vi "Dashboard Main.vi"() -> ()   [LabVIEW 2013]
uses:
  <vilib>/event_ctls.llb/eventvkey.ctl
  <vilib>/Rock Robotics/WPI/Dashboard/WPI_DashboardLogging Global.vi
  <vilib>/Utility/config.llb/Write Key (String).vi
  <vilib>/Utility/config.llb/Write Key (I32).vi
  <vilib>/Utility/config.llb/NI_LVConfig.lvlib
panel:
  out "Image Message":string="Timeout in Camera Communications"
  in  "Rec Mode":enum32{"Stop", "Record", "Playback"}(radio)
  in  "Dashboard Tab":T1(tab)
  in  "Camera Settings":T2={"Frame Rate"=30, "Compression"=30, "Size"=1} {"Frame Rate" scale=1.0..30.0; "Size" items=["640x480", "320x240", "160x120"]}
  out "MotorSliders R":cluster{"MotorSlide1":dbl, "MotorSlide2":dbl} {"MotorSlide2" scale=-1.0..1.0 scale format="%#_2e"; "MotorSlide1" scale=-1.0..1.0 scale format="%#_2e"}
  out "MotorChart R":cluster{"Numeric":dbl, "Numeric":dbl}(graph)
  out "MotorSliders L":T3 {"MotorSlide4 2" scale=0.0..14.0 scale format="%#_2e"; "MotorSlide2" scale=-1.0..1.0 scale format="%#_2e"; "MotorSlide1" scale=-1.0..1.0 scale format="%#_2e"}
  out "MotorChart L":T4(graph)
  out "JS1 Z":dbl(slide) scale=-1.0..1.0 scale format="%#_2e"
  out "Joystick 1":cluster{"X":dbl, "Y":dbl}[](graph)
  out "JS Buttons 1":T5
  out "JS2 Z":dbl(slide) scale=-1.0..1.0 scale format="%#_2e"
  out "Joystick 2":cluster{"X":dbl, "Y":dbl}[](graph)
  out "JS Buttons 2":T5
  out "Mode":T6(ring)=enum."Auto Disabled"
  out "Camera IP":string
  in  "DB Camera Config":bool
  out "fps":dbl format="%#.1g"
  out "Mbps":dbl format="%#.1g"
  out "Mbps 2":bool
  out "LED 1":bool
  out "Tanks Full":bool
  in  "Compressor On":bool
  out "Compression Pressure":dbl(slide) scale=0.0..10.0
  in  "Slider 1":dbl(slide) scale=0.0..100.0
  in  "Checkbox 2":bool
  in  "Checkbox 1":bool
  in  "Test Slider":dbl(slide) scale=0.0..100.0 scale format="%#_3g"
  in  "On/Off":bool caption="Solenoid"
  in  "Test Name":u16(ring) items=["Select the test to run...", "Example Test", "-------------------------------", "List of tests is built in robot code.", "Replace with your own automated tests."]
  in  "Test Tree":string(tree)
  in  "Motor":cluster{"Value":dbl, "Enable":bool} {"Value" scale=-1.0..1.0 scale format="%#_3g"}
  out "Progress":T7 {"Test Progress" scale=0.0..100.0}
  in  "Rev/Fwd":cluster{"Forward":bool, "Reverse":bool}
  in  "Test Ring":u16(ring) items=["Auto", "Fixed indoor", "Fixed outdoor 1", "Fixed outdoor 2", "Fixed fluorescent 1", "Fixed fluorescent 2", "Hold current"]
  in  "Listbox":i32(listbox)
  out "Tree":string(tree)
  out "Camera Image":T8(plugin-control)
  in  "Enable":bool
  # "Left"
  # "Front"
  # "Right"
  # "Battery"
  # "Customize by placing controls and indicators here and name to\nmatch Dashboard Variables on robot."
  # "This tab is a great place for autonomous settings and validation.\nCustomize by placing controls and indicators here and name to\nmatch Dashboard Variables on robot."
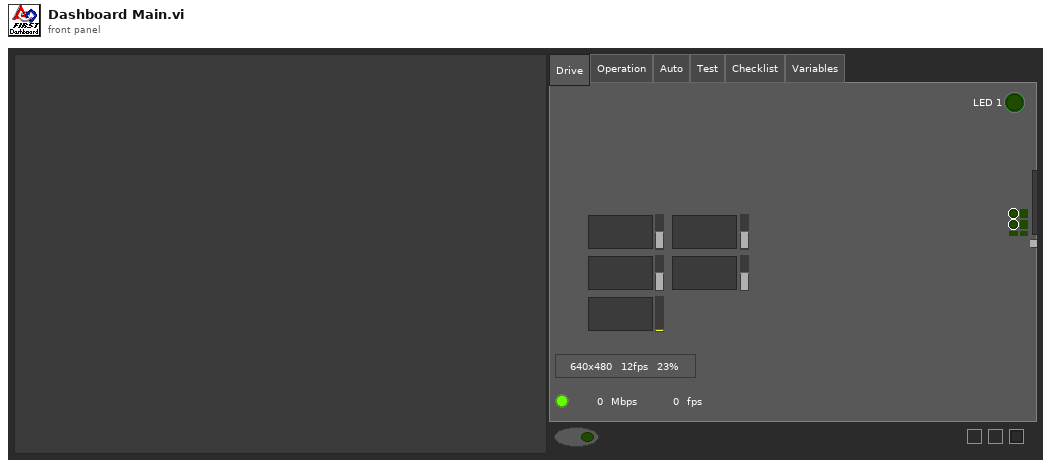
[diagram p1: front panel]
types:
  T1 = enum32{"Drive", "Operation", "Auto", "Test", "Checklist", "Variables"}
  T2 = cluster{"Frame Rate":i32, "Compression":i32, "Size":u16}
  T3 = cluster{"MotorSlide1":dbl, "MotorSlide2":dbl, "MotorSlide4 2":dbl}
  T4 = cluster{"Numeric":dbl, "Numeric":dbl, "Battery":sgl}
  T5 = cluster{bool, bool, bool, bool, bool, bool, bool, bool, bool, bool, bool, bool}
  T6 = enum8{"Tele-Op Disabled", "Tele-Op Enabled", "Auto Disabled", "Auto Enabled", "Test Disabled", "Test Enabled", ""}
  T7 = cluster{"Test Progress":u8, "Test Progress Text":string}
  T8 = typedef "IMAQ Image.ctl" = refnum<image>
  T9 = typedef "Image Type" = u32
  T10 = cluster{"Digital Inputs":bool[], "Digital Outputs":bool[]}
  T11 = cluster{"Competition mode":bool, "Robot Link":bool, "Autonomous":bool, "Enabled":bool, "E-Stop":bool, "Simulated":bool, "TestMode":bool, "Docked Window":bool}
  T12 = cluster{"Boolean Array[0]":bool, "Boolean Array[1]":bool, "Boolean Array[2]":bool, "Boolean Array[3]":bool, "Boolean Array[4]":bool, "Boolean Array[5]":bool, "Boolean Array[6]":bool, "Boolean Array[7]":bool, "Boolean Array[8]":bool, "Boolean Array[9]":bool, "Boolean Array[10]":bool, "Boolean Array[11]":bool}
  T13 = typedef "NI_LVConfig.lvlib/Config Data RefNum.ctl" = refnum<k1>
  T14 = typedef "eventvkey.ctl" = enum16{"ASCII", "Enter", "Return", "Shift", "Ctrl", "Alt", "Cmd", "Opt", "Caps", "NumLock", "Clear", "Break", "Up", "Down", "Left", "Right", "Insert", "Delete", "Home", "End", "PageUp", "PageDown", "Escape", "Help", "Pause", "ScrollLock", "F1", "F2", "F3", "F4", "F5", "F6", "F7", "F8", "F9", "F10", "F11", "F12", "F13", "F14", "F15", "F16", "F17", "F18", "F19", "F20", "F21", "F22", "F23", "F24", "Play", "VolumeUp", "VolumeDown", "Mute", "Two Byte Char"}
  T15 = cluster{"Image Size":bool, "Image Type":bool, "Pixel Value":bool, "ROI Information":bool, "Zoom Factor":bool}
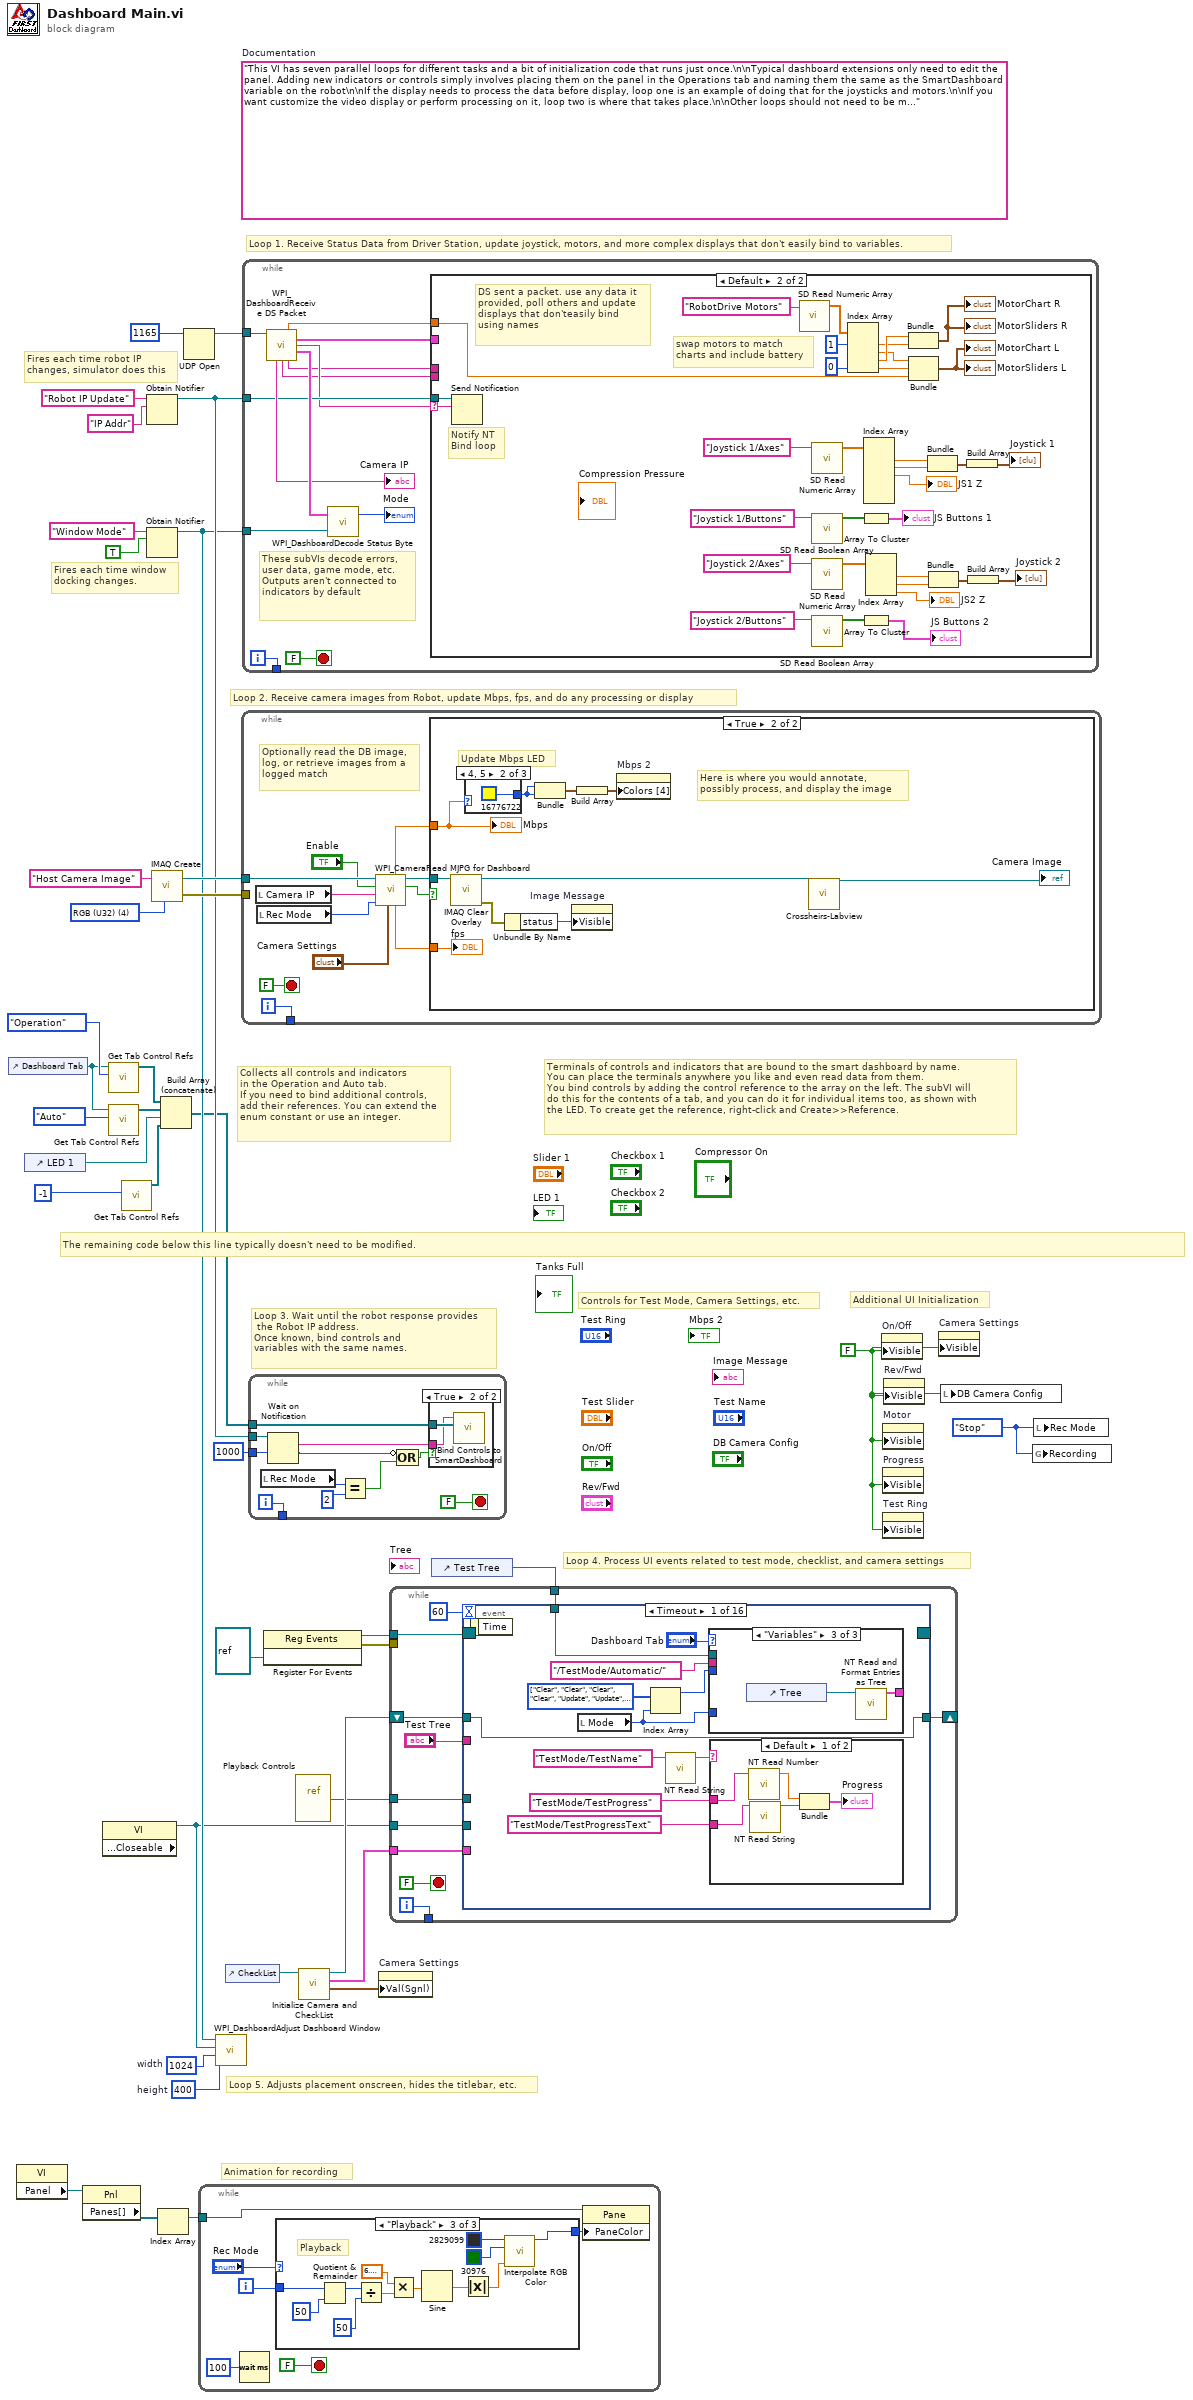
[diagram p0: block diagram]
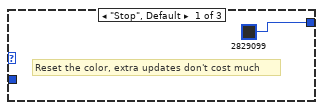
[diagram p2: hidden frame]
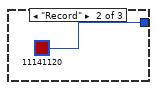
[diagram p3: hidden frame]
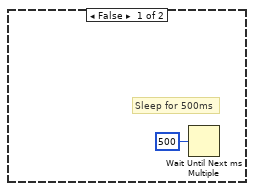
[diagram p5: hidden frame]
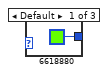
[diagram p6: hidden frame]
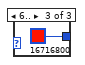
[diagram p7: hidden frame]
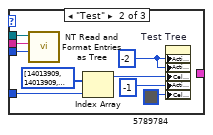
[diagram p9: hidden frame]
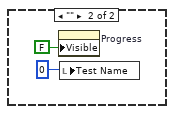
[diagram p10: hidden frame]
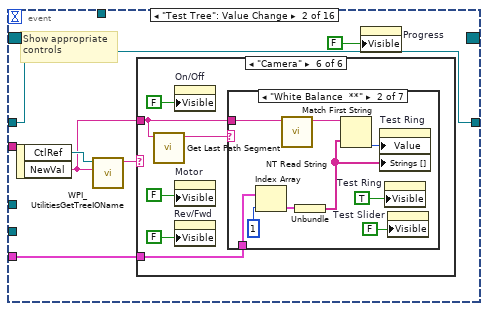
[diagram p11: hidden frame]
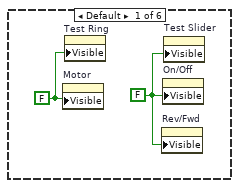
[diagram p12: hidden frame]
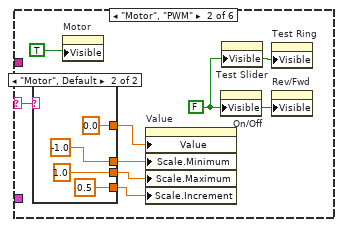
[diagram p13: hidden frame]
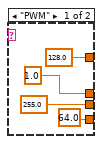
[diagram p14: hidden frame]
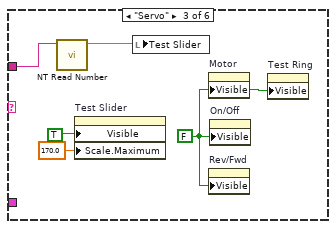
[diagram p15: hidden frame]
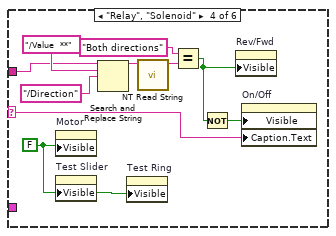
[diagram p16: hidden frame]
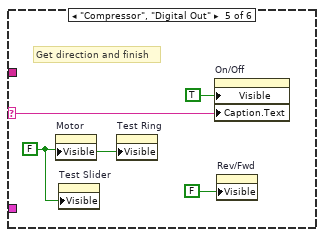
[diagram p17: hidden frame]
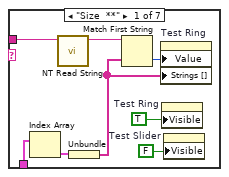
[diagram p18: hidden frame]
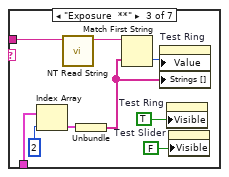
[diagram p19: hidden frame]
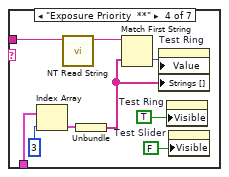
[diagram p20: hidden frame]
diagram:
  w10 = enum32{"Stop", "Record", "Playback"}."Stop" ("Rec Mode")
  w13 = 400  # height
  w14 = 1024  # width
  w27 = FALSE ("Visible")
  (unwired) "This VI has seven parallel loops for different tasks and a bit of initialization code that runs just once.\n\nTypical dashboard extensions only need to edit the panel. Adding new indicators or controls simply involves placing them on the panel in the Operations tab and naming them the same as the SmartDashboard variable on the robot\n\nIf the display needs to process the data before display, loop one is an example of doing that for the joysticks and motors.\n\nIf you want customize the video display or perform processing on it, loop two is where that takes place.\n\nOther loops should not need to be modified. They are pretty standard, and document the task they perform."  # Documentation
  w37 = T9 4 items=["Grayscale (U8)", "Grayscale (I16)", "Grayscale (SGL)", "Complex (CSG)", "RGB (U32)", "HSL (U32)", "RGB (U64)"] ("Image Type")
  # "Controls for Test Mode, Camera Settings, etc."
  # "Additional UI Initialization"
  # "Animation for recording"
  # "Fires each time robot IP\nchanges, simulator does this"
  # "Fires each time window\ndocking changes."
  # "Collects all controls and indicators\nin the Operation and Auto tab.\nIf you need to bind additional controls,\nadd their references. You can extend the\nenum constant or use an integer."
  # "The remaining code below this line typically doesn't need to be modified."
  # "Loop 4. Process UI events related to test mode, checklist, and camera settings"
  # "Terminals of controls and indicators that are bound to the smart dashboard by name.\nYou can place the terminals anywhere you like and even read data from them.\nYou bind controls by adding the control reference to the array on the left. The subVI will\ndo this for the contents of a tab, and you can do it for individual items too, as shown with\nthe LED. To create get the reference, right-click and Create>>Reference."
  # "Loop 3. Wait until the robot response provides\n the Robot IP address.\nOnce known, bind controls and\nvariables with the same names."
  # "Loop 5. Adjusts placement onscreen, hides the titlebar, etc."
  # "Loop 1. Receive Status Data from Driver Station, update joystick, motors, and more complex displays that don't easily bind to variables."
  # "Loop 2. Receive camera images from Robot, update Mbps, fps, and do any processing or display"
  n1 = control-ref of="Dashboard Tab"() -> (w8:refnum<vi>)
  n2 = property class="VI"() -> ("Panel"=w21:refnum<vi>)  [unwired: 2 in, 2 out]
  n3 = control-ref of="LED 1"() -> (w3:refnum<vi>)
  n4 = property class="Pnl"(reference=w21) -> ("Panes[]"=w22:refnum<vi>[])  [unwired: 1 in, 2 out]
  n5 = property class="VI" props=["Front Panel.Closeable"]() -> (reference out=w9:refnum<vi>)  [unwired: 2 in, 2 out]
  n6 = call <vilib>:"Get Tab Control Refs.vi"("Page Index"=T1."Operation" ("Dashboard Tab"), "TabControl in"=w8) -> ("ControlsOnPage"=w6:refnum<vi>[])  [unwired: 9 in]
  n7 = call <vilib>:"Get Tab Control Refs.vi"("Page Index"=T1."Auto" ("Dashboard Tab"), "TabControl in"=w8) -> ("ControlsOnPage"=w7:refnum<vi>[])  [unwired: 9 in]
  n8 = call <vilib>:"Get Tab Control Refs.vi"("Page Index"=-1) -> ("ControlsOnPage"=w2:refnum<vi>[])  [unwired: 10 in]
  n9 = Obtain Notifier(name (unnamed)="Robot IP Update", notification data type="IP Addr" ("name (unnamed)")) -> (notifier out=w31:refnum<notifier>)  [unwired: 2 in, 2 out]
  n10 = Obtain Notifier(name (unnamed)="Window Mode", notification data type=TRUE) -> (notifier out=w12:refnum<notifier>)  [unwired: 2 in, 2 out]
  n11 = call "IMAQ Create"("Image Name"="Host Camera Image", "Image Type"=w37) -> ("New Image"=w35:T8, "error out"=w34:errorcluster)  [unwired: 2 in, 1 out]
  n12 = Index Array(array=w22) -> (element=w20:refnum<vi>)  [unwired: 1 in]
  n13 = Build Array (concatenate)(w6, w7, w3, w2) -> (w5:refnum<vi>[])
  n14 = UDP Open(11:u16 1165 ("port")) -> (port=w38:refnum<k16>)  [unwired: 2 in, 4 out]
  n15 = while {
    tunnel: w20 -> [w41]
    i -> [w44]
    stop <- FALSE stop-if-true
    n16 = Wait (ms)(milliseconds to wait=u32 100) -> ()  [unwired: 1 out]
    n17 = case shown="\"Playback\"" "Rec Mode" {
      tunnel: w44 -> [_ _ w59]
      tunnel: [u32 2829099 ("Base Color") u32 11141120 ("Target Color") w48] -> w40
      frame "Stop", Default {
        # "Reset the color, extra updates don't cost much"
      }
      frame "Record" {
      }
      frame "Playback" {
        # "Playback"
        n18 = Quotient & Remainder(x=w59, y=u32 50 ("milliseconds to wait")) -> (x-y*floor(x/y)=w55:u32)  [unwired: 1 out]
        n19 = Divide(x=w55, y=u32 50 ("milliseconds to wait")) -> (x/y=w52:dbl)
        n20 = Multiply(x=6.283185307179586, y=w52) -> (x*y=w57:dbl)
        n21 = Sine(x=w57) -> (sin(x)=w56:dbl)
        n22 = Absolute Value(x=w56) -> (abs(x)=w49:dbl)
        n23 = call "Interpolate RGB Color.vi"("Proportion"=w49, "Target Color"=u32 30976, "Base Color"=u32 2829099) -> ("Result Color"=w48:u32)  [unwired: 8 in]
      }
    }
    n24 = property class="Pane"(reference=w41, "PaneColor"=w40) -> ()  [unwired: 1 in, 2 out]
  }
  n25 = call <vilib>:"WPI_DashboardAdjust Dashboard Window.vi"("height"=w13, "width"=w14, "reference in"=w9, "Notifier in"=w12) -> ()  [unwired: 8 in]
  n26 = control-ref of="CheckList"() -> (w11:refnum<vi>)
  n27 = while {
    tunnel: w35 -> [w68]
    tunnel: w34 -> [_]
    tunnel: [w69] -> _
    i -> [w69]
    stop <- FALSE stop-if-true
    # "Optionally read the DB image,\nlog, or retrieve images from a\nlogged match"
    n28 = local read "Camera IP"() -> (w61:string)
    n29 = local read "Rec Mode"() -> (w60:enum32{"Stop", "Record", "Playback"})
    n30 = call <vilib>:"WPI_CameraRead MJPG for Dashboard.vi"("Camera Settings"="Camera Settings", "Rec Mode"=w60, "Camera IP"=w61, "Enable"="Enable", "Refnum in"=w68) -> ("Active"=w65:bool, "Refnum out"=w67:T8, "FPS"=w64:dbl, "Bandwidth (Mbps)"=w63:dbl)  [unwired: 3 in]
    n31 = case shown="True" w65 {
      tunnel: w67 -> [_ w76]
      tunnel: w63 -> [_ w75]
      tunnel: w64 -> [_ w74]
      frame False {
        # "Sleep for 500ms"
        n32 = Wait Until Next ms Multiple(millisecond multiple=u32 500) -> ()  [unwired: 1 out]
      }
      frame True {
        # "Here is where you would annotate,\npossibly process, and display the image"
        # "Update Mbps LED"
        n33 = call "IMAQ Clear Overlay"("Image"=w76) -> ("error out"=w80:errorcluster, "Image Out"=w73:T8)  [unwired: 2 in, 7 out]
        n34 = case shown="4, 5" w75 {
          tunnel: [u32 6618880 ("Color Box") u32 16776722 ("Color Box") u32 16716800 ("Color Box")] -> w77
          frame Default {
          }
          frame 4, 5 {
          }
          frame 6.. {
          }
        }
        n35 = Unbundle By Name(w80) -> ("status"=w81:bool)
        n36 = Bundle("Color Box"=w77, "Color Box"=w77) -> (w79:cluster{"Color Box":u32, "Color Box":u32})  [unwired: 1 out]
        n37 = property on="Image Message" class="Str"("Visible"=w81) -> ()  [unwired: 2 in, 2 out]
        n38 = Build Array(w79) -> (w78:cluster{"Color Box":u32, "Color Box":u32}[])
        n39 = property on="Mbps 2" class="Bool (strict)"("Colors [4]"=w78) -> ()  [unwired: 2 in, 2 out]
        n40 = call "Crossheirs-Labview.vi"("Image In"=w73) -> ("Image Out"=→"Camera Image":T8)  [unwired: 25 in, 1 out]
        "Mbps" <- w75
        "fps" <- w74
      }
    }
  }
  n41 = while {
    tunnel: w38 -> [w95]
    tunnel: w31 -> [w90]
    tunnel: w12 -> [w94]
    tunnel: [w91] -> _
    i -> [w91]
    stop <- FALSE stop-if-true
    # "These subVIs decode errors, user data, game mode, etc.\nOutputs aren't connected to indicators by default"
    n42 = call <vilib>:"WPI_DashboardReceive DS Packet.vi"("Recv Socket"=w95) -> ("Battery"=w85:sgl, "Driver Station"=w86:T10, "Robot IP Address"=w89:string, "Status"=w96:T11, "Camera IP Address"=→"Camera IP":string, "Low Priority User Data"=w88:string, "High Priority User Data"=w87:string)  [unwired: 1 in, 7 out]
    n43 = call <vilib>:"WPI_DashboardDecode Status Byte.vi"("Window Mode Notifier"=w94, "Status"=w96) -> ("Mode"=→"Mode":T6)  [unwired: 1 out]
    n44 = case shown="Default" w89 {
      selector: w89 -> [_ w108]
      tunnel: w90 -> [_ w109]
      tunnel: w88 -> [_ _]
      tunnel: w87 -> [_ _]
      tunnel: w86 -> [_ _]
      tunnel: w85 -> [_ w107]
      frame "0.0.0.0" {
        # "DS not sending packets, or no robot exists yet.\nDon't poll the variables"
      }
      frame Default {
        # "Notify NT\nBind loop"
        # "DS sent a packet. use any data it\nprovided, poll others and update\ndisplays that don'teasily bind\nusing names"
        # "swap motors to match\ncharts and include battery"
        n45 = Send Notification(notification=w108, notifier=w109) -> ()  [unwired: 1 in, 2 out]
        n46 = call <vilib>:"SD Read Numeric Array.vi"("Name"="RobotDrive Motors") -> ("Numeric Array"=w106:dbl[])  [unwired: 8 in, 2 out]
        n47 = call <vilib>:"SD Read Numeric Array.vi"("Name"="Joystick 1/Axes") -> ("Numeric Array"=w125:dbl[])  [unwired: 8 in, 2 out]
        n48 = call <vilib>:"SD Read Boolean Array.vi"("Name"="Joystick 1/Buttons") -> ("Boolean Array"=w127:bool[])  [unwired: 8 in, 2 out]
        n49 = call <vilib>:"SD Read Numeric Array.vi"("Name"="Joystick 2/Axes") -> ("Numeric Array"=w119:dbl[])  [unwired: 8 in, 2 out]
        n50 = call <vilib>:"SD Read Boolean Array.vi"("Name"="Joystick 2/Buttons") -> ("Boolean Array"=w118:bool[])  [unwired: 8 in, 2 out]
        n51 = Index Array(array=w106, index #1=1, index #4=0) -> (element #1=w102:dbl, element #2=w101:dbl, element #3=w103:dbl, element #4=w98:dbl)  [unwired: 2 in]
        n52 = Array To Cluster(array=w127) -> (cluster=→"JS Buttons 1":T12)
        n53 = Array To Cluster(array=w118) -> (cluster=→"JS Buttons 2":T12)
        n54 = Index Array(array=w125) -> (element #1=w122:dbl, element #2=w123:dbl, element #3=→"JS1 Z":dbl)  [unwired: 6 in, 3 out]
        n55 = Index Array(array=w119) -> (element #1=w114:dbl, element #2=w113:dbl, element #3=→"JS2 Z":dbl)  [unwired: 3 in]
        n56 = Bundle("Numeric"=w103, "Numeric"=w102) -> (→"MotorChart R" →"MotorSliders R":cluster{"Numeric":dbl, "Numeric":dbl})  [unwired: 1 in]
        n57 = Bundle("Numeric"=w101, "Numeric"=w98, "Battery"=w107) -> (→"MotorChart L" →"MotorSliders L":T4)  [unwired: 1 in]
        n58 = Bundle("Numeric"=w122, "Numeric"=w123) -> (w121:cluster{"Numeric":dbl, "Numeric":dbl})  [unwired: 1 in]
        n59 = Bundle("Numeric"=w114, "Numeric"=w113) -> (w115:cluster{"Numeric":dbl, "Numeric":dbl})  [unwired: 1 in]
        n60 = Build Array(w121) -> (→"Joystick 1":cluster{"Numeric":dbl, "Numeric":dbl}[])
        n61 = Build Array(w115) -> (→"Joystick 2":cluster{"Numeric":dbl, "Numeric":dbl}[])
      }
    }
  }
  n62 = while {
    tunnel: w5 -> [w141]
    tunnel: w31 -> [w139]
    tunnel: [w137] -> _
    tunnel: u32 1000 ("milliseconds to wait") -> [w136]
    i -> [w137]
    stop <- FALSE stop-if-true
    n63 = local read "Rec Mode"() -> (w132:enum32{"Stop", "Record", "Playback"})
    n64 = Wait on Notification(notifier=w139, timeout in ms (-1)=w136) -> (notification=w138:string, timed out?=w134:bool)  [unwired: 2 in, 2 out]
    n65 = Equal?(x=w132, y=u16 2 ("Rec Mode")) -> (x = y?=w133:bool)
    n66 = Compound Arithmetic op=OR(invert w134, w133) -> (w135:bool)
    n67 = case shown="True" w135 {
      tunnel: w141 -> [_ w143]
      tunnel: w138 -> [_ w142]
      frame False {
      }
      frame True {
        n68 = call <vilib>:"Bind Controls to SmartDashboard.vi"("Bound Control Refs"=w143, "Server IP Address"=w142) -> ()  [unwired: 10 in]
      }
    }
  }
  n69 = register-events(refnum<vi> refnum) -> (reference out=w18:refnum<event-registration>, error out=w17:errorcluster)  [unwired: 2 in]
  n70 = vi-ref "Playback Controls.vi"() -> (w19:refnum<vi>)
  n71 = call "Initialize Camera and CheckList.vi"("ListBox in"=w11) -> ("Cluster"=w25:cluster{"value":i32, "value":i32, "index":i32}, "Array"=w26:cluster{string[]}[], "File Refnum"=w24:T13)  [unwired: 8 in]
  n72 = property on="Camera Settings" class="Clust (strict)"("Val(Sgnl)"=w25) -> ()  [unwired: 2 in, 2 out]
  n73 = control-ref of="Test Tree"() -> (w23:refnum<vi>)
  n74 = while {
    tunnel: w26 -> [w151]
    shift-right: [w150] -> _
    shift-left: w24 -> [w149]
    tunnel: [w148] -> _
    tunnel: w23 -> [w147]
    tunnel: w19 -> [w146]
    tunnel: w18 -> [w145]
    tunnel: w17 -> [_]
    tunnel: w9 -> [w144]
    i -> [w148]
    stop <- FALSE stop-if-true
    n75 = event shown="[0] Timeout" {
      selector: w145 -> [_ _ _ _ _ _ _ _ _ _ _ _ _ _ _ _]
      dyn-events: [_ _ _ _ _ _ _ _ _ _ _ _ _ w389 _ _] -> _
      timeout: u32 60 ("milliseconds to wait") -> [_ _ _ _ _ _ _ _ _ _ _ _ _ _ _ _]
      tunnel: w147 -> [w161 _ _ _ _ _ _ _ _ _ _ _ _ _ _ _]
      tunnel: "Test Tree" -> [_ _ _ _ _ _ _ _ w358 w366 w368 w372 w380 _ _ _]
      tunnel: w151 -> [_ w185 _ _ _ _ w322 w352 _ _ _ _ _ _ _ _]
      tunnel: [w155 w184 w283 w288 w296 w308 w321 w345 w357 w364 w367 w371 w379 w391 w405 w406] -> w150
      tunnel: w149 -> [w155 w184 w283 w288 w296 w308 w320 w345 w357 w364 w367 w371 w379 w391 w405 w406]
      tunnel: w146 -> [_ _ _ _ _ _ _ _ _ _ _ _ _ w392 _ w409]
      tunnel: w144 -> [_ _ _ _ _ _ _ _ _ _ _ _ _ w387 _ _]
      event Timeout {
        w160 = enum16{"Update", "Clear"}[] [enum."Clear", enum."Clear", enum."Clear", enum."Clear", enum."Update", enum."Update", enum."Clear"] items=["Update", "Clear"]
        n76 = event-data() -> ()  [unwired: 1 in, 1 out]
        n77 = local read "Mode"() -> (w158:T6)
        n78 = Index Array(array=w160, index=w158) -> (element=w159:enum16{"Update", "Clear"})
        n79 = call <vilib>:"NT Read String.vi"("Name"="TestMode/TestName") -> ("String"=w164:string)  [unwired: 9 in, 1 out]
        n80 = case shown="\"Variables\"" "Dashboard Tab" {
          tunnel: w161 -> [_ w174 _]
          tunnel: "/TestMode/Automatic/" ("Name Pattern") -> [_ w173 _]
          tunnel: w159 -> [_ w172 _]
          tunnel: w158 -> [_ w170 _]
          tunnel: [_ _ w176] -> _
          frame "Operation", Default {
          }
          frame "Test" {
            w169 = -2 ("Active Item:Row Number")
            n81 = call <vilib>:"NT Read and Format Entries as Tree.vi"("Operation"=w172, "Name Pattern"=w173, "Tree Refnum"=w174) -> ()  [unwired: 7 in, 2 out]
            n82 = Index Array(array=u32[] [14013909, 14013909, 14013909, 14013909, 14013909, 16777215, 14013909], index=w170) -> (element=w168:u32)
            n83 = property on="Test Tree" class="Tree (strict)"("Active Item Row Number"=w169, "ActiveColNum"=w169, "CellBG"=w168, "Active Item Row Number"=-1 ("Active Item:Row Number"), "CellBG"=u32 5789784 ("Color Box")) -> ()  [unwired: 2 in, 2 out]
          }
          frame "Variables" {
            n84 = control-ref of="Tree"() -> (w175:refnum<vi>)
            n85 = call <vilib>:"NT Read and Format Entries as Tree.vi"("Tree Refnum"=w175) -> ("Formatted Strings"=w176:cluster{"Name":string, "Value":string}[])  [unwired: 9 in, 1 out]
          }
        }
        n86 = case shown="Default" w164 {
          tunnel: "TestMode/TestProgress" ("Name") -> [w178 _]
          tunnel: "TestMode/TestProgressText" ("Name") -> [w177 _]
          frame Default {
            n87 = call <vilib>:"NT Read Number.vi"("Name"=w178) -> ("Numeric"=w179:dbl)  [unwired: 9 in, 1 out]
            n88 = call <vilib>:"NT Read String.vi"("Name"=w177) -> ("String"=w180:string)  [unwired: 9 in, 1 out]
            n89 = Bundle("Numeric"=w179, "String"=w180) -> (→"Progress":cluster{"Numeric":dbl, "String":string})  [unwired: 1 in]
          }
          frame "" {
            n90 = property on="Progress" class="Clust (strict)"("Visible"=FALSE) -> ()  [unwired: 2 in, 2 out]
            n91 = local write "Test Name"(u16 0) -> ()
          }
        }
      }
      event "Test Tree": Value Change {
        # "Show appropriate\ncontrols"
        n92 = event-data() -> ("CtlRef"=w188:refnum<vi>, "NewVal"=w186:string)  [unwired: 1 in]
        n93 = call <vilib>:"WPI_UtilitiesGetTreeIOName.vi"("NewVal"=w186, "TreeControl in"=w188) -> ("I/O Name"=w189:string)  [unwired: 9 in]
        n94 = case shown="\"Camera\"" w189 {
          selector: w189 -> [_ w196 _ w214 w223 _]
          tunnel: w186 -> [_ _ w211 w213 _ w230]
          tunnel: w185 -> [_ _ _ _ _ w229]
          frame Default {
            w191 = FALSE ("Visible")
            w190 = FALSE ("Visible")
            n95 = property on="Motor" class="Clust (strict)"("Visible"=w190) -> ()  [unwired: 2 in, 2 out]
            n96 = property on="Test Ring" class="Ring (strict)"("Visible"=w190) -> ()  [unwired: 2 in, 2 out]
            n97 = property on="Rev/Fwd" class="Clust (strict)"("Visible"=w191) -> ()  [unwired: 2 in, 2 out]
            n98 = property on="On/Off" class="Bool (strict)"("Visible"=w191) -> ()  [unwired: 2 in, 2 out]
            n99 = property on="Test Slider" class="Slide (strict)"("Visible"=w191) -> ()  [unwired: 2 in, 2 out]
          }
          frame "Motor", "PWM" {
            w197 = FALSE ("Visible")
            n100 = case shown="\"Motor\", Default" w196 {
              tunnel: [1.0 ("Value") -1.0 ("Value")] -> w195
              tunnel: [255.0 ("Value") 1.0 ("Value")] -> w194
              tunnel: [128.0 ("Value") 0.0 ("Value")] -> w193
              tunnel: [64.0 ("Value") 0.5 ("Value")] -> w192
              frame "PWM" {
              }
              frame "Motor", Default {
              }
            }
            n101 = property on="Motor" class="Clust (strict)"("Visible"=TRUE) -> ()  [unwired: 2 in, 2 out]
            n102 = property on="Value" class="Slide (strict)"("Value"=w193, "Scale.Minimum"=w195, "Scale.Maximum"=w194, "Scale.Increment"=w192) -> ()  [unwired: 2 in, 2 out]
            n103 = property on="On/Off" class="Bool (strict)"("Visible"=w197) -> ()  [unwired: 2 in, 2 out]
            n104 = property on="Test Slider" class="Slide (strict)"("Visible"=w197) -> ()  [unwired: 2 in, 2 out]
            n105 = property on="Test Ring" class="Ring (strict)"("Visible"=w197) -> ()  [unwired: 2 in, 2 out]
            n106 = property on="Rev/Fwd" class="Clust (strict)"("Visible"=w197) -> ()  [unwired: 2 in, 2 out]
          }
          frame "Servo" {
            w209 = FALSE ("Visible")
            n107 = call <vilib>:"NT Read Number.vi"("Name"=w211) -> ("Numeric"=w210:dbl)  [unwired: 9 in, 1 out]
            n108 = property on="Test Slider" class="Slide (strict)"("Visible"=TRUE, "Scale.Maximum"=170.0 ("Scale.Range:Maximum")) -> ()  [unwired: 2 in, 2 out]
            n109 = local write "Test Slider"(w210) -> ()
            n110 = property on="Motor" class="Clust (strict)"("Visible"=w209) -> ()  [unwired: 2 in, 2 out]
            n111 = property on="Rev/Fwd" class="Clust (strict)"("Visible"=w209) -> ()  [unwired: 2 in, 2 out]
            n112 = property on="On/Off" class="Bool (strict)"("Visible"=w209) -> ()  [unwired: 2 in, 2 out]
            n113 = property on="Test Ring" class="Ring (strict)"("Visible"=w209) -> ()  [unwired: 2 in, 2 out]
          }
          frame "Relay", "Solenoid" {
            w212 = FALSE ("Visible")
            n114 = property on="Motor" class="Clust (strict)"("Visible"=w212) -> ()  [unwired: 2 in, 2 out]
            n115 = property on="Test Slider" class="Slide (strict)"("Visible"=w212) -> ()  [unwired: 2 in, 2 out]
            n116 = Search and Replace String(input string=w213, search string="/Value  **", replace string="/Direction") -> (result string=w219:string)  [unwired: 5 in, 3 out]
            n117 = property on="Test Ring" class="Ring (strict)"("Visible"=w212) -> ()  [unwired: 2 in, 2 out]
            n118 = call <vilib>:"NT Read String.vi"("Name"=w219) -> ("String"=w217:string)  [unwired: 9 in, 1 out]
            n119 = Equal?(x="Both directions", y=w217) -> (x = y?=w215:bool)
            n120 = Not(x=w215) -> (.not. x?=w216:bool)
            n121 = property on="Rev/Fwd" class="Clust (strict)"("Visible"=w215) -> ()  [unwired: 2 in, 2 out]
            n122 = property on="On/Off" class="Bool (strict)"("Visible"=w216, "Caption.Text"=w214) -> ()  [unwired: 2 in, 2 out]
          }
          frame "Compressor", "Digital Out" {
            w222 = FALSE ("Visible")
            # "Get direction and finish"
            n123 = property on="Motor" class="Clust (strict)"("Visible"=w222) -> ()  [unwired: 2 in, 2 out]
            n124 = property on="Test Slider" class="Slide (strict)"("Visible"=w222) -> ()  [unwired: 2 in, 2 out]
            n125 = property on="Test Ring" class="Ring (strict)"("Visible"=w222) -> ()  [unwired: 2 in, 2 out]
            n126 = property on="On/Off" class="Bool (strict)"("Visible"=TRUE, "Caption.Text"=w223) -> ()  [unwired: 2 in, 2 out]
            n127 = property on="Rev/Fwd" class="Clust (strict)"("Visible"=FALSE) -> ()  [unwired: 2 in, 2 out]
          }
          frame "Camera" {
            n128 = call <vilib>:"Get Last Path Segment.vi"("String in"=w230) -> ("String out"=w231:string)  [unwired: 10 in]
            n129 = property on="On/Off" class="Bool (strict)"("Visible"=FALSE) -> ()  [unwired: 2 in, 2 out]
            n130 = property on="Motor" class="Clust (strict)"("Visible"=FALSE) -> ()  [unwired: 2 in, 2 out]
            n131 = property on="Rev/Fwd" class="Clust (strict)"("Visible"=FALSE) -> ()  [unwired: 2 in, 2 out]
            n132 = case shown="\"White Balance  **\"" w231 {
              tunnel: w230 -> [w237 w246 w255 w264 w273 _ w279]
              tunnel: w229 -> [w235 w243 w252 w261 w270 _ _]
              frame "Size  **" {
                n133 = Index Array(array=w235) -> (element=w234:cluster{string[]})  [unwired: 1 in]
                n134 = call <vilib>:"NT Read String.vi"("Name"=w237) -> ("String"=w236:string)  [unwired: 9 in, 1 out]
                n135 = Unbundle(w234) -> (w232:string[])
                n136 = Match First String(2:w232, 3:w236) -> (0:w233:i32)  [unwired: 1 out]
                n137 = property on="Test Ring" class="Ring (strict)"("Value"=w233, "Strings []"=w232) -> ()  [unwired: 2 in, 2 out]
                n138 = property on="Test Ring" class="Ring (strict)"("Visible"=TRUE) -> ()  [unwired: 2 in, 2 out]
                n139 = property on="Test Slider" class="Slide (strict)"("Visible"=FALSE) -> ()  [unwired: 2 in, 2 out]
              }
              frame "White Balance  **" {
                n140 = Index Array(array=w243, index=1) -> (element=w244:cluster{string[]})
                n141 = call <vilib>:"NT Read String.vi"("Name"=w246) -> ("String"=w245:string)  [unwired: 9 in, 1 out]
                n142 = Unbundle(w244) -> (w241:string[])
                n143 = Match First String(2:w241, 3:w245) -> (0:w240:i32)  [unwired: 1 out]
                n144 = property on="Test Ring" class="Ring (strict)"("Value"=w240, "Strings []"=w241) -> ()  [unwired: 2 in, 2 out]
                n145 = property on="Test Ring" class="Ring (strict)"("Visible"=TRUE) -> ()  [unwired: 2 in, 2 out]
                n146 = property on="Test Slider" class="Slide (strict)"("Visible"=FALSE) -> ()  [unwired: 2 in, 2 out]
              }
              frame "Exposure  **" {
                n147 = Index Array(array=w252, index=2) -> (element=w253:cluster{string[]})
                n148 = call <vilib>:"NT Read String.vi"("Name"=w255) -> ("String"=w254:string)  [unwired: 9 in, 1 out]
                n149 = Unbundle(w253) -> (w249:string[])
                n150 = Match First String(2:w249, 3:w254) -> (0:w250:i32)  [unwired: 1 out]
                n151 = property on="Test Ring" class="Ring (strict)"("Value"=w250, "Strings []"=w249) -> ()  [unwired: 2 in, 2 out]
                n152 = property on="Test Ring" class="Ring (strict)"("Visible"=TRUE) -> ()  [unwired: 2 in, 2 out]
                n153 = property on="Test Slider" class="Slide (strict)"("Visible"=FALSE) -> ()  [unwired: 2 in, 2 out]
              }
              frame "Exposure Priority  **" {
                n154 = Index Array(array=w261, index=3) -> (element=w262:cluster{string[]})
                n155 = call <vilib>:"NT Read String.vi"("Name"=w264) -> ("String"=w263:string)  [unwired: 9 in, 1 out]
                n156 = Unbundle(w262) -> (w258:string[])
                n157 = Match First String(2:w258, 3:w263) -> (0:w259:i32)  [unwired: 1 out]
                n158 = property on="Test Ring" class="Ring (strict)"("Value"=w259, "Strings []"=w258) -> ()  [unwired: 2 in, 2 out]
                n159 = property on="Test Ring" class="Ring (strict)"("Visible"=TRUE) -> ()  [unwired: 2 in, 2 out]
                n160 = property on="Test Slider" class="Slide (strict)"("Visible"=FALSE) -> ()  [unwired: 2 in, 2 out]
              }
              frame "Color Enable  **" {
                n161 = Index Array(array=w270, index=4) -> (element=w271:cluster{string[]})
                n162 = call <vilib>:"NT Read String.vi"("Name"=w273) -> ("String"=w272:string)  [unwired: 9 in, 1 out]
                n163 = Unbundle(w271) -> (w267:string[])
                n164 = Match First String(2:w267, 3:w272) -> (0:w268:i32)  [unwired: 1 out]
                n165 = property on="Test Ring" class="Ring (strict)"("Value"=w268, "Strings []"=w267) -> ()  [unwired: 2 in, 2 out]
                n166 = property on="Test Ring" class="Ring (strict)"("Visible"=TRUE) -> ()  [unwired: 2 in, 2 out]
                n167 = property on="Test Slider" class="Slide (strict)"("Visible"=FALSE) -> ()  [unwired: 2 in, 2 out]
              }
              frame Default {
                n168 = property on="Test Ring" class="Ring (strict)"("Visible"=FALSE) -> ()  [unwired: 2 in, 2 out]
                n169 = property on="Test Slider" class="Slide (strict)"("Visible"=FALSE) -> ()  [unwired: 2 in, 2 out]
              }
              frame "Brightness  **", "Color Level  **", "Compression  **", "FPS  **", "Sharpness  **" {
                n170 = call <vilib>:"NT Read Number.vi"("Name"=w279) -> ("Numeric"=w278:dbl)  [unwired: 9 in, 1 out]
                n171 = local write "Test Slider"(w278) -> ()
                n172 = property on="Test Slider" class="Slide (strict)"("Visible"=TRUE, "Scale.Maximum"=100.0 ("Scale.Range:Maximum")) -> ()  [unwired: 2 in, 2 out]
                n173 = property on="Test Ring" class="Ring (strict)"("Visible"=FALSE) -> ()  [unwired: 2 in, 2 out]
              }
            }
          }
        }
        n174 = property on="Progress" class="Clust (strict)"("Visible"=FALSE) -> ()  [unwired: 2 in, 2 out]
      }
      event "Test Name": Mouse Enter {
        # "Populate the ring with the list of tests"
        n175 = event-data() -> ()  [unwired: 1 in, 1 out]
        n176 = call <vilib>:"NT Read String Array.vi"("Name"="TestMode/TestList") -> ("String Array"=w287:string[])  [unwired: 9 in, 1 out]
        n177 = Build Array (concatenate)("Select the test to run...", w287) -> (w286:string[])
        n178 = property on="Test Name" class="Ring (strict)"("Strings []"=w286) -> ()  [unwired: 2 in, 2 out]
      }
      event "Test Name": Value Change {
        w289 = FALSE ("Visible")
        # "Tell the robot the test name to run"
        n179 = event-data() -> ("NewVal"=w293:u16)  [unwired: 1 in]
        n180 = property on="Test Name" class="Ring (strict)"() -> ("Strings []"=w294:string[])  [unwired: 2 in, 2 out]
        n181 = local write "Progress"(T7 {"Test Progress"=0, "Test Progress Text"=""} ("Progress")) -> ()
        n182 = Index Array(array=w294, index=w293) -> (element=w292:string)
        n183 = call <vilib>:"NT Write String.vi"("String"=w292, "Name"="TestMode/TestName") -> ()  [unwired: 9 in, 1 out]
        n184 = property on="Progress" class="Clust (strict)"("Visible"=TRUE) -> ()  [unwired: 2 in, 2 out]
        n185 = property on="Motor" class="Clust (strict)"("Visible"=w289) -> ()  [unwired: 2 in, 2 out]
        n186 = property on="Test Slider" class="Slide (strict)"("Visible"=w289) -> ()  [unwired: 2 in, 2 out]
        n187 = property on="On/Off" class="Bool (strict)"("Visible"=w289) -> ()  [unwired: 2 in, 2 out]
        n188 = property on="Rev/Fwd" class="Clust (strict)"("Visible"=w289) -> ()  [unwired: 2 in, 2 out]
        n189 = property on="Test Ring" class="Ring (strict)"("Visible"=w289) -> ()  [unwired: 2 in, 2 out]
      }
      event "Listbox": Double Click {
        n190 = event-data() -> ("PlatMods.Shift"=w297:bool, "Row"=w299:i32)  [unwired: 1 in]
        n191 = case shown="True" w297 {
          tunnel: w299 -> [w303 _]
          tunnel: 1 -> [w302 _]
          frame False {
            n192 = property on="Listbox" class="LstBox (strict)"() -> ("Item Symbols"=w301:i32[])  [unwired: 2 in, 2 out]
            n193 = Replace Array Subset(array=w301, new element=w302, index=w303) -> (w300:i32[])
            n194 = property on="Listbox" class="LstBox (strict)"("Item Symbols"=w300) -> ()  [unwired: 2 in, 2 out]
          }
          frame True {
            w304 = 0 ("Top Row")
            n195 = property on="Listbox" class="LstBox (strict)"() -> ("Number of Rows"=w306:u32)  [unwired: 2 in, 2 out]
            n196 = Initialize Array(0, w306) -> (w305:i32[])
            n197 = property on="Listbox" class="LstBox (strict)"("Top Row"=w304, "Value"=w304, "Item Symbols"=w305) -> ()  [unwired: 2 in, 2 out]
          }
        }
      }
      event "Listbox": Key Down {
        n198 = event-data() -> ("VKey"=w310:T14)  [unwired: 1 in]
        n199 = case shown="\"Left\", \"Right\"" w310 {
          selector: w310 -> [w315 _]
          tunnel: eventvkey."Left" ("VKey") -> [w313 _]
          frame "Left", "Right" {
            n200 = Equal?(x=w313, y=w315) -> (x = y?=w314:bool)
            n201 = Select(t=0, s=w314, f=1) -> (s? t:f=w316:i32)
            n202 = property on="Listbox" class="LstBox (strict)"() -> ("Item Symbols"=w319:i32[])  [unwired: 2 in, 2 out]
            n203 = Replace Array Subset(array=w319, new element=w316, index="Listbox") -> (w318:i32[])
            n204 = property on="Listbox" class="LstBox (strict)"("Item Symbols"=w318) -> ()  [unwired: 2 in, 2 out]
          }
          frame Default {
          }
        }
      }
      event "DB Camera Config": Value Change {
        n205 = event-data() -> ("NewVal"=w323:bool)  [unwired: 1 in]
        n206 = case shown="False" w323 {
          tunnel: w322 -> [w332 _]
          tunnel: [w325 w343] -> w321
          tunnel: w320 -> [w324 w343]
          frame False {
            w339 = "Camera"
            w342 = FALSE ("Visible")
            n207 = local read "Camera Settings"() -> (w331:T2)
            n208 = Index Array(array=w332) -> (element=w335:cluster{string[]})  [unwired: 1 in]
            n209 = Unbundle(w331) -> ("Frame Rate"=w330:i32, "Compression"=w329:i32, "Size"=w333:u16)
            n210 = Unbundle(w335) -> (w334:string[])
            n211 = Index Array(array=w334, index=w333) -> (element=w328:string)
            n212 = call-poly <vilib>:"Write Key.vi"("section"=w339, "value"=w328, "key"="Size", "refnum"=w324) -> ("refnum out"=w341:T13)  [unwired: 2 in, 5 out]
            n213 = call-poly <vilib>:"Write Key.vi"("section"=w339, "value"=w330, "key"="FrameRate", "refnum"=w341) -> ("refnum out"=w340:T13)  [unwired: 1 in, 6 out]
            n214 = property on="Camera Settings" class="Clust (strict)"("Visible"=w342) -> ()  [unwired: 2 in, 2 out]
            n215 = local write "DB Camera Config"(w342) -> ()
            n216 = call-poly <vilib>:"Write Key.vi"("section"=w339, "value"=w329, "key"="Compression", "refnum"=w340) -> ("refnum out"=w326:T13)  [unwired: 1 in, 6 out]
            n217 = call <vilib>:"Close Config Data.vi"("refnum"=w326) -> ("file path"=w327:path)  [unwired: 2 in, 8 out]
            n218 = call <vilib>:"Open Config Data.vi"("configuration file path"=w327) -> ("refnum"=w325:T13)  [unwired: 8 in, 2 out]
          }
          frame True {
            n219 = property on="Camera Settings" class="Clust (strict)"("Visible"=TRUE) -> ()  [unwired: 2 in, 2 out]
          }
        }
      }
      event "Camera Settings": Value Change {
        n220 = event-data() -> ("NewVal"=w356:T2)  [unwired: 1 in]
        n221 = Index Array(array=w352) -> (element=w351:cluster{string[]})  [unwired: 1 in]
        n222 = Unbundle(w356) -> ("Frame Rate"=w347:i32, "Compression"=w346:i32, "Size"=w349:u16)
        n223 = Unbundle(w351) -> (w350:string[])
        n224 = Index Array(array=w350, index=w349) -> (element=w348:string)
        n225 = Format Into String(format string="%s   %dfps   %d%%", w348, w347, w346) -> (resulting string=w353:string)  [unwired: 2 in, 1 out]
        n226 = Build Array(w353) -> (w354:string[])
        n227 = property on="DB Camera Config" class="Bool (strict)"("Strings [4]"=w354) -> ()  [unwired: 2 in, 2 out]
      }
      event "Motor.Enable": Value Change {
        n228 = event-data() -> ("NewVal"=w362:bool)  [unwired: 1 in]
        n229 = Unbundle("Motor") -> ("Value"=w361:dbl)  [unwired: 1 out]
        n230 = Select(t=w361, s=w362, f=0.0) -> (s? t:f=w359:dbl)
        n231 = call <vilib>:"NT Write Number.vi"("Numeric"=w359, "Name"=w358) -> ()  [unwired: 9 in, 1 out]
      }
      event "Test Slider": Value Change {
        n232 = event-data() -> ("NewVal"=w365:dbl)  [unwired: 1 in]
        n233 = call <vilib>:"NT Write Number.vi"("Numeric"=w365, "Name"=w366) -> ()  [unwired: 9 in, 1 out]
      }
      event "On/Off": Value Change {
        n234 = event-data() -> ("NewVal"=w370:bool)  [unwired: 1 in]
        n235 = Boolean To (0,1)(Boolean=w370) -> (0, 1=w369:i16)
        n236 = call <vilib>:"NT Write Number.vi"("Numeric"=w369, "Name"=w368) -> ()  [unwired: 9 in, 1 out]
      }
      event "Rev/Fwd": Value Change {
        n237 = event-data() -> ("NewVal.Forward"=w378:bool, "NewVal.Reverse"=w377:bool)  [unwired: 1 in]
        n238 = Boolean To (0,1)(Boolean=w378) -> (0, 1=w374:i16)
        n239 = Boolean To (0,1)(Boolean=w377) -> (0, 1=w376:i16)
        n240 = Negate(x=w376) -> (-x=w375:i16)
        n241 = Add(x=w374, y=w375) -> (x+y=w373:i16)
        n242 = call <vilib>:"NT Write Number.vi"("Numeric"=w373, "Name"=w372) -> ()  [unwired: 9 in, 1 out]
      }
      event "Test Ring": Value Change {
        n243 = event-data() -> ("NewVal"=w382:u16)  [unwired: 1 in]
        n244 = property on="Test Ring" class="Ring (strict)"() -> ("Strings []"=w383:string[])  [unwired: 2 in, 2 out]
        n245 = Index Array(array=w383, index=w382) -> (element=w381:string)
        n246 = call <vilib>:"NT Write String.vi"("String"=w381, "Name"=w380) -> ()  [unwired: 9 in, 1 out]
      }
      event "Rec Mode": Value Change {
        # "Update globals for recording mode and path to read log from.\nClear when logging and let NetworkTables set path for vision to\nuse."
        n247 = event-data() -> ("NewVal"=w393:enum32{"Stop", "Record", "Playback"})  [unwired: 1 in]
        n248 = global write "WPI_DashboardLogging Global.vi" "Logging Filename"(path "") -> ()
        n249 = case shown="\"Stop\", \"Record\"" w393 {
          tunnel: w392 -> [_ w395 w403]
          tunnel: [_ _ w402] -> w389
          tunnel: [_ _ w401] -> _
          tunnel: w387 -> [_ _ w399]
          tunnel: cluster{i32, i32} {-250, 170} -> [_ _ w398]
          tunnel: [_ _ T15 {"Image Size"=TRUE, "Image Type"=TRUE, "Pixel Value"=TRUE, "ROI Information"=TRUE, "Zoom Factor"=FALSE} ("Image Information Shown:All Elements")] -> w385
          tunnel: [_ _ TRUE ("Zoom Factor")] -> w384
          frame Default {
          }
          frame "Stop", "Record" {
            # "Place Window too"
            n250 = invoke class="VI" method="FP.Close"(reference=w395) -> (reference out=w394:refnum<vi>)  [unwired: 2 in, 2 out]
            n251 = invoke class="VI" method="Abort VI"(reference=w394) -> ()  [unwired: 2 in, 3 out]
          }
          frame "Playback" {
            n252 = call "Open Playback Panel.vi"("Offset"=w398, "DB VI Ref"=w399, "Playback in"=w403) -> ("Playback out"=w400:refnum<vi>)  [unwired: 8 in]
            n253 = register-events(w400) -> (reference out=w402:refnum<event-registration>, error out=w401:errorcluster)  [unwired: 2 in]
          }
        }
        n254 = global write "WPI_DashboardLogging Global.vi" "Recording"(w393) -> ()
        n255 = property on="Camera Image" class="ImageControl"("Image Information Shown"=w385, "Image Information Visible"=w384) -> ()  [unwired: 2 in, 2 out]
        n256 = call <vilib>:"WPI_DashboardNT Log FieldName Cache.vi"("Operation"=enum16{"Lookup/Add", "Index", "Clear"}."Clear") -> ()  [unwired: 8 in, 3 out]
      }
      event Panel Close {
        w404 = enum32{"Stop", "Record", "Playback"}."Stop" ("Rec Mode")
        n257 = event-data() -> ()  [unwired: 1 in, 4 out]
        n258 = local write "Rec Mode"(w404) -> ()
        n259 = global write "WPI_DashboardLogging Global.vi" "Recording"(w404) -> ()
      }
      event Panel Close {
        # "Abort playback window and ourself"
        n260 = event-data() -> ()  [unwired: 1 in, 4 out]
        n261 = invoke class="VI" method="FP.Close"(reference=w409) -> (reference out=w408:refnum<vi>)  [unwired: 2 in, 2 out]
        n262 = invoke class="VI" method="Abort VI"(reference=w408) -> (error out=w407:errorcluster)  [unwired: 2 in, 2 out]
        n263 = invoke class="VI" method="Abort VI"(error in=w407) -> ()  [unwired: 2 in, 3 out]
      }
    }
  }
  n264 = property on="On/Off" class="Bool (strict)"("Visible"=w27) -> ()  [unwired: 2 in, 2 out]
  n265 = property on="Motor" class="Clust (strict)"("Visible"=w27) -> ()  [unwired: 2 in, 2 out]
  n266 = property on="Progress" class="Clust (strict)"("Visible"=w27) -> ()  [unwired: 2 in, 2 out]
  n267 = property on="Test Ring" class="Ring (strict)"("Visible"=w27) -> ()  [unwired: 2 in, 2 out]
  n268 = property on="Rev/Fwd" class="Clust (strict)"("Visible"=w27) -> ()  [unwired: 2 in, 2 out]
  n269 = property on="Camera Settings" class="Clust (strict)"("Visible"=w27) -> ()  [unwired: 2 in, 2 out]
  n270 = local write "DB Camera Config"(w27) -> ()
  n271 = global write "WPI_DashboardLogging Global.vi" "Recording"(w10) -> ()
  n272 = local write "Rec Mode"(w10) -> ()
